vi "DL-Parse Waveforms.vi"(0 "Waveform array":waveform(dbl)[](array[waveform])) -> (4 "timestamp":dbl, 8 "2D Array":dbl[][](array[numeric]))   [LabVIEW 2020]
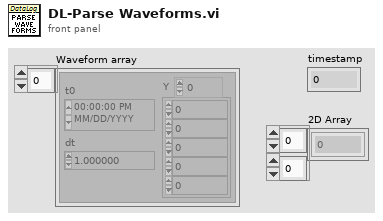
[diagram p1: front panel]
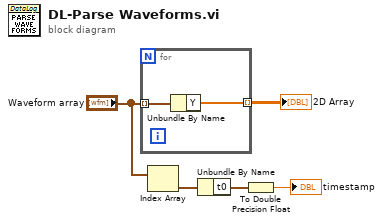
[diagram p0: block diagram]
diagram:
  n1 = for {
    tunnel: "Waveform array" -> [w7] mode=indexing
    tunnel: [w6] -> w5 mode=indexing
    n2 = Unbundle By Name(w7) -> ("Y"=w6:dbl[])
  }
  "2D Array" <- w5
  n3 = Index Array(array="Waveform array") -> (element=w3:waveform(dbl))  [unwired: 1 in]
  n4 = Unbundle By Name(w3) -> ("t0"=w2:timestamp)
  n5 = To Double Precision Float(number=w2) -> (double precision float=→"timestamp":dbl)
